vi "多影像平均.vi"() -> ()   [LabVIEW 2015]
uses:
  <vilib>/vision/NI_Vision_Development_Module.lvlib
panel:
  out "Image_array":T1[](array[plugin-control])
  in  "stop":bool
  in  "Horizontal Progress Bar":u8(slide) scale=0.0..255.0
  out "Threshole_array":T1[](array[plugin-control])
  out "Waveform Graph 3":T2(graph)
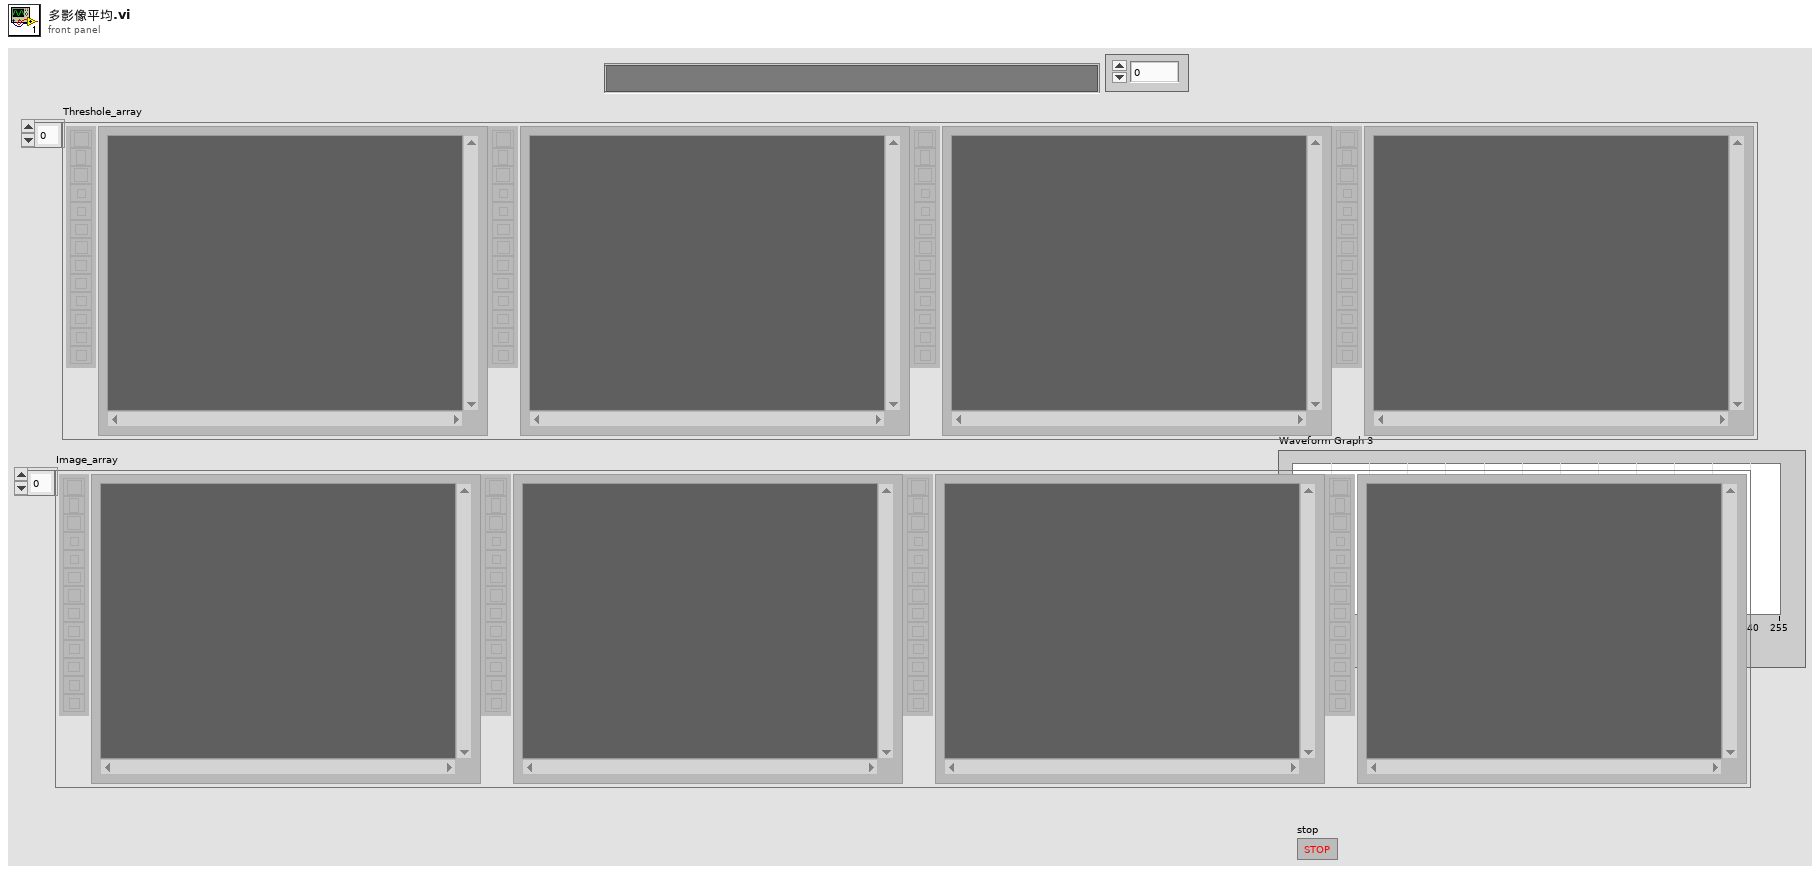
[diagram p1: front panel]
types:
  T1 = typedef "IMAQ Image.ctl" = refnum<image>
  T2 = cluster{"Starting Value":sgl, "Incremental Value":sgl, "Histogram":u32[]}[]
  T3 = typedef "Image Type" = u32
  T4 = cluster{"Starting Value":sgl, "Incremental Value":sgl, "Histogram":u32[]}
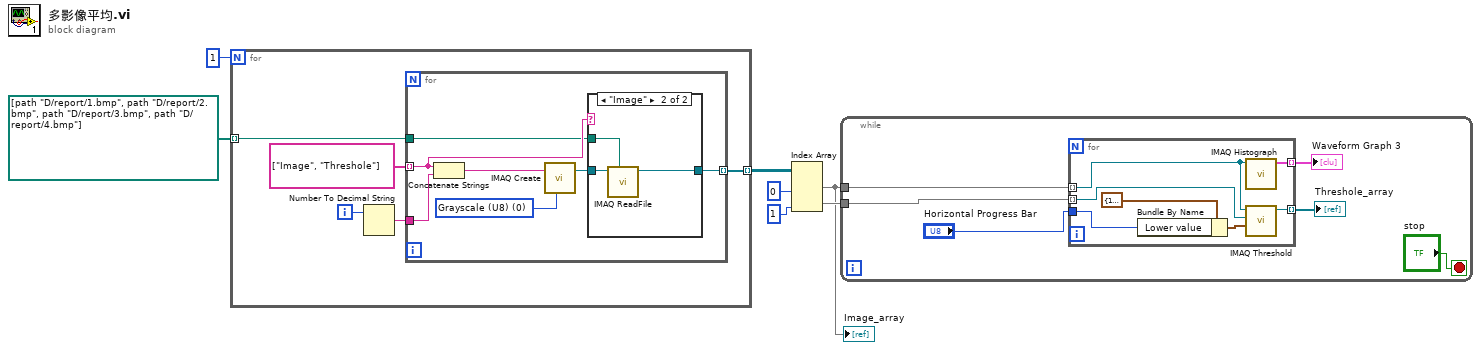
[diagram p0: block diagram]
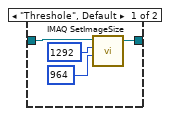
[diagram p2: hidden frame]
diagram:
  n1 = for {
    N: 1 -> [_]
    tunnel: [w9] -> w3 mode=indexing
    tunnel: path[] [path "D:/report/1.bmp", path "D:/report/2.bmp", path "D:/report/3.bmp", path "D:/report/4.bmp"] -> [w8] mode=indexing
    i -> [w12]
    n2 = Number To Decimal String(number=w12) -> (decimal integer string=w10:string)  [unwired: 1 in]
    n3 = for {
      tunnel: string[] ["Image", "Threshole"] -> [w16] mode=indexing
      tunnel: w10 -> [w18]
      tunnel: [w14] -> w9 mode=indexing
      tunnel: w8 -> [w13]
      w19 = T3 0 items=["Grayscale (U8)", "Grayscale (I16)", "Grayscale (SGL)", "Complex (CSG)", "RGB (U32)", "HSL (U32)", "RGB (U64)", "Grayscale (U16)"] ("Image Type")
      n4 = Concatenate Strings(w16, w18) -> (w17:string)
      n5 = call "IMAQ Create"("Image Name"=w17, "Image Type"=w19) -> ("New Image"=w15:T1)  [unwired: 3 in, 1 out]
      n6 = case shown="\"Image\"" w16 {
        tunnel: w15 -> [w21 w26]
        tunnel: [w20 w25] -> w14
        tunnel: w13 -> [_ w24]
        frame "Threshole", Default {
          n7 = call "IMAQ SetImageSize"("Y Resolution"=964, "X Resolution"=1292, "Image"=w21) -> ("Image Out"=w20:T1)  [unwired: 2 in, 1 out]
        }
        frame "Image" {
          n8 = call "IMAQ ReadFile"("File Path"=w24, "Image"=w26) -> ("Image Out"=w25:T1)  [unwired: 5 in, 4 out]
        }
      }
    }
  }
  n9 = Index Array(array=w3, index (col) #1=0 ("index (row)"), index (col) #2=1 ("index (row)")) -> (element #1=w1:T1[], element #2=w6:T1[])  [unwired: 2 in]
  "Image_array" <- w1
  n10 = while {
    tunnel: w6 -> [w30]
    tunnel: w1 -> [w27]
    stop <- "stop" stop-if-true
    n11 = for {
      tunnel: w27 -> [w39] mode=indexing
      tunnel: w30 -> [w38] mode=indexing
      tunnel: [w37] -> w31 mode=indexing
      tunnel: [w34] -> w29 mode=indexing
      tunnel: "Horizontal Progress Bar" -> [w33]
      n12 = Bundle By Name(cluster=cluster{"Lower value":sgl, "Upper value":sgl} {"Lower value"=128.0, "Upper value"=255.0} ("Range"), "Lower value"=w33) -> (w35:cluster{"Lower value":sgl, "Upper value":sgl})
      n13 = call "IMAQ Histograph"("Image"=w39) -> ("Histogram Graph"=w34:T4)  [unwired: 7 in, 3 out]
      n14 = call "IMAQ Threshold"("Range"=w35, "Image Dst"=w38, "Image Src"=w39) -> ("Image Dst Out"=w37:T1)  [unwired: 7 in, 1 out]
    }
    "Threshole_array" <- w31
    "Waveform Graph 3" <- w29
  }
